vi "Measurement Plugin File Names.vi"() -> (6 "Get Type Specializations":string)   [LabVIEW 2020, in "MeasurementLink Measurement Server.lvlib"]
uses:
  MeasurementLink Measurement Server.lvlib
panel:
  # "TODO: Consider instead a single polymorphic VI with a single string output"
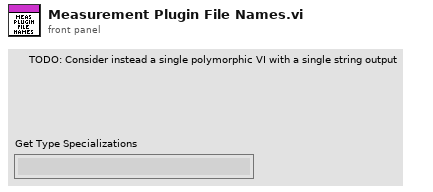
[diagram p1: front panel]
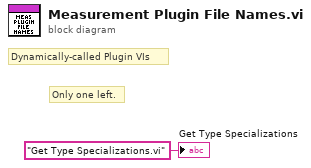
[diagram p0: block diagram]
diagram:
  # "Only one left."
  # "Dynamically-called Plugin VIs"
  "Get Type Specializations" <- "Get Type Specializations.vi" ("Get Measurement Details")
